vi "FlatToRichrfcontrol_RangeResponse.vi"(5 "OutputClusterType":T1, 11 "InputCluster":T2) -> (3 "OutputCluster":T1)   [LabVIEW 2024, in "FlexSDR_gRPC_client.lvlib"]
uses:
  FlexSDR_gRPC_client.lvlib
  rfcontrol_RangeResponse_Flat.ctl
  rfcontrol_RangeResponse.ctl
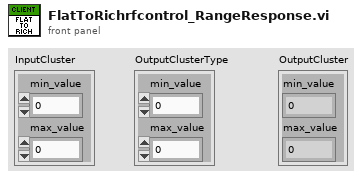
[diagram p1: front panel]
types:
  T1 = typedef "FlexSDR_gRPC_client.lvlib/rfcontrol_RangeResponse.ctl" = cluster{"min_value":dbl, "max_value":dbl}
  T2 = typedef "FlexSDR_gRPC_client.lvlib/rfcontrol_RangeResponse_Flat.ctl" = cluster{"min_value":dbl, "max_value":dbl}
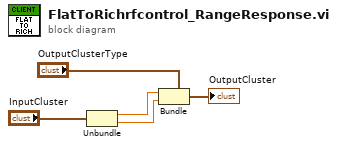
[diagram p0: block diagram]
diagram:
  n1 = Unbundle "Unbundle"("InputCluster") -> ("min_value"=w2:dbl, "max_value"=w1:dbl)
  n2 = Bundle "Bundle"(cluster="OutputClusterType", "min_value"=w2, "max_value"=w1) -> (→"OutputCluster":T1)
